vi "test_Basic Write and Read.vi"(8 "error in (no error)":errorcluster, 11 "Scalar Channels Testing in":refnum<class "FPGA Addon Test Class.lvclass">) -> (0 "error out":errorcluster, 3 "Scalar Channels Testing out":refnum<class "FPGA Addon Test Class.lvclass">)   [LabVIEW 2019]
uses:
  FPGA Addon Test Class.lvclass
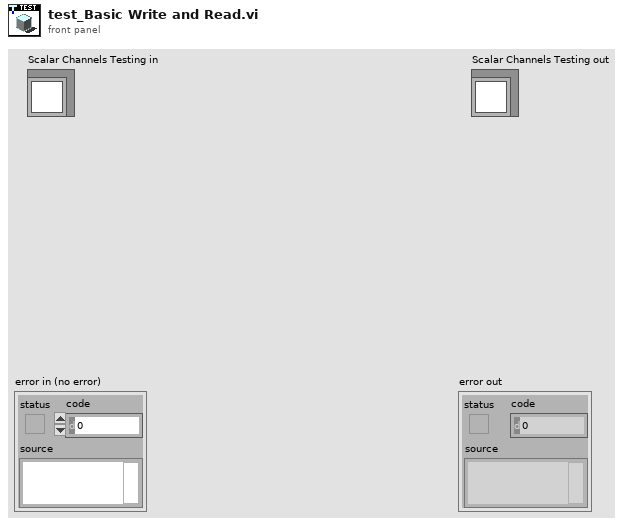
[diagram p1: front panel]
types:
  T1 = typedef "NI_VS Workspace ExecutionAPI.lvlib/WorkspaceAPI.ctl" = refnum<k24>
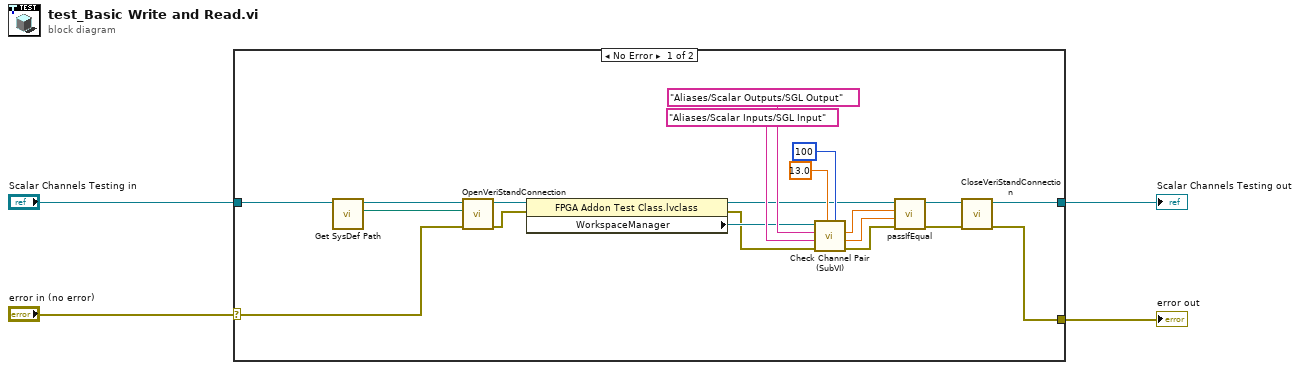
[diagram p0: block diagram]
diagram:
  n1 = case shown="No Error" "error in (no error)" {
    selector: "error in (no error)" -> [w5 w26]
    tunnel: [w23 w26] -> w3
    tunnel: [w24 w25] -> w1
    tunnel: "Scalar Channels Testing in" -> [w8 w25]
    frame No Error {
      n2 = call "Get SysDef Path.vi"("Scalar Channels Testing in"=w8) -> ("SysDef Path"=w6:path, "Scalar Channels Testing out"=w7:refnum<class "FPGA Addon Test Class.lvclass">)  [unwired: 9 in]
      n3 = call-dynamic "OpenVeriStandConnection.vi"("error in (no error)"=w5, "System Definition File"=w6, "VeriStand Test Case in"=w7) -> ("error out"=w18:errorcluster, "VeriStand Test Case out"=w17:refnum<class "FPGA Addon Test Class.lvclass">)  [unwired: 6 in, 1 out]
      n4 = property class="FPGA Addon Test Class.lvclass"(reference=w17, error in=w18) -> (reference out=w14:refnum<class "FPGA Addon Test Class.lvclass">, error out=w15:errorcluster, "WorkspaceManager"=w16:T1)
      n5 = call "Check Channel Pair (SubVI).vi"("milliseconds to wait"=u32 100, "Test Value"=13.0 ("Value"), "error in (no error)"=w15, "Input Channel"="Aliases/Scalar Inputs/SGL Input" ("Channel"), "Output Channel"="Aliases/Scalar Outputs/SGL Output" ("Channel"), "WorkspaceManager in"=w16) -> ("error out"=w10:errorcluster, "InputChannel Value"=w12:dbl, "OutputChannel Value"=w13:dbl)  [unwired: 2 in, 1 out]
      n6 = call-dynamic "passIfEqual.vi"("error in (no error)"=w10, "y"=w12, "x"=w13, "TestCase in"=w14) -> ("error out"=w9:errorcluster, "TestCase out"=w11:refnum<class "FPGA Addon Test Class.lvclass">)  [unwired: 6 in]
      n7 = call-dynamic "CloseVeriStandConnection.vi"("error in (no error)"=w9, "VeriStand Test Case in"=w11) -> ("error out"=w23:errorcluster, "VeriStand Test Case out"=w24:refnum<class "FPGA Addon Test Class.lvclass">)  [unwired: 8 in]
    }
    frame Error {
    }
  }
  "error out" <- w3
  "Scalar Channels Testing out" <- w1
